vi "FlexQueryTicklish.vi"(9 "write buffer":string, 11 "Serial USB port name":refnum<visa-resource-name>) -> (0 "error out":errorcluster, 1 "Result string":string, 3 "Serial USB port name out":refnum<visa-resource-name>)   [LabVIEW 2015]
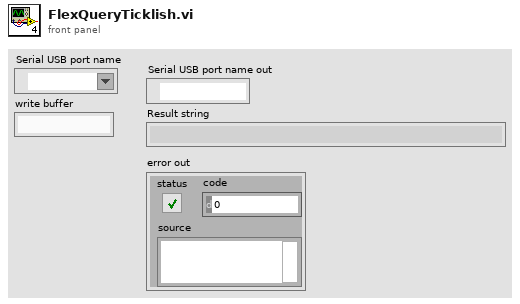
[diagram p1: front panel]
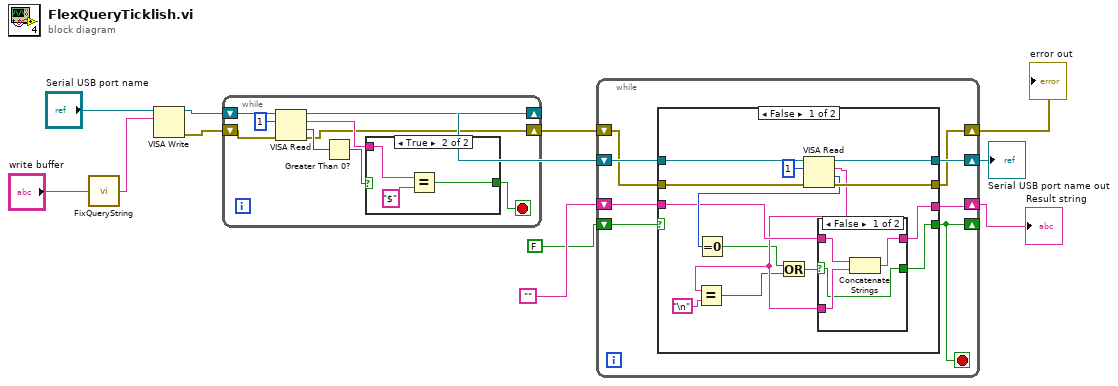
[diagram p0: block diagram]
diagram:
  n1 = call "FixQueryString.vi"("write buffer"="write buffer") -> ("write buffer fixed"=w1:string)  [unwired: 4 in]
  n2 = VISA Write(VISA resource name="Serial USB port name", write buffer=w1) -> (VISA resource name out=w11:refnum<visa-resource-name>, error out=w10:errorcluster)  [unwired: 1 in, 1 out]
  n3 = while {
    shift-right: [w20] -> w9
    shift-left: w11 -> [w21]
    shift-right: [w13] -> w8
    shift-left: w10 -> [w14]
    stop <- w15 stop-if-true
    n4 = VISA Read(VISA resource name=w21, byte count=u32 1, error in (no error)=w14) -> (VISA resource name out=w20:refnum<visa-resource-name>, read buffer=w16:string, return count=w18:u32, error out=w13:errorcluster)
    n5 = Greater Than 0?(x=w18) -> (x > 0?=w17:bool)
    n6 = case shown="True" w17 {
      selector: w17 -> [w22 _]
      tunnel: w16 -> [_ w25]
      tunnel: [w22 w23] -> w15
      frame False {
      }
      frame True {
        n7 = Equal?(x=w25, y="$") -> (x = y?=w23:bool)
      }
    }
  }
  n8 = while {
    shift-right: [w32] -> w6
    shift-left: w9 -> [w33]
    shift-right: [w30] -> w4
    shift-left: w8 -> [w31]
    shift-right: [w28] -> w5
    shift-left: "" -> [w29]
    shift-right: [w26] -> _
    shift-left: FALSE -> [w27]
    stop <- w26 stop-if-true
    n9 = case shown="False" w27 {
      selector: w27 -> [_ w57]
      tunnel: [w41 w57] -> w26
      tunnel: w33 -> [w47 w56]
      tunnel: [w46 w56] -> w32
      tunnel: w31 -> [w44 w55]
      tunnel: [w43 w55] -> w30
      tunnel: w29 -> [w40 w54]
      tunnel: [w39 w54] -> w28
      frame False {
        n10 = VISA Read(VISA resource name=w47, byte count=u32 1, error in (no error)=w44) -> (VISA resource name out=w46:refnum<visa-resource-name>, read buffer=w38:string, return count=w42:u32, error out=w43:errorcluster)
        n11 = Equal?(x=w38, y="\n") -> (x = y?=w34:bool)
        n12 = Equal To 0?(x=w42) -> (x = 0?=w35:bool)
        n13 = Or(x=w35, y=w34) -> (x .or. y?=w36:bool)
        n14 = case shown="False" w36 {
          selector: w36 -> [w48 w53]
          tunnel: [w48 w53] -> w41
          tunnel: w40 -> [w50 w52]
          tunnel: [w49 w52] -> w39
          tunnel: w38 -> [w51 _]
          frame False {
            n15 = Concatenate Strings(w50, w51) -> (w49:string)
          }
          frame True {
          }
        }
      }
      frame True {
      }
    }
  }
  "Serial USB port name out" <- w6
  "Result string" <- w5
  "error out" <- w4
